vi "_LC Get Status.vi"(8 "Stream#":u8) -> (0 "error out":errorcluster, 1 "Error":bool, 2 "Ready":bool, 3 "LC Status":string, 4 "StatusIndicator":u16(ring)=1 caption="Status Indicator")   [LabVIEW 2015]
uses:
  Type/_LC Command.ctl
  _Global LC Driver.vi
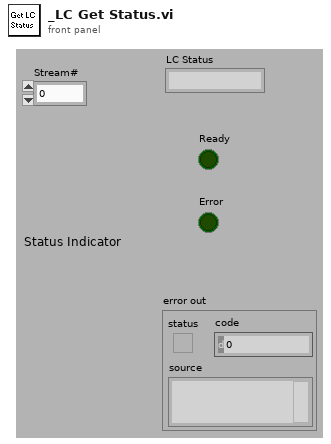
[diagram p1: front panel]
types:
  T1 = typedef "_LC Command.ctl" = enum16{"No Command", "Initialize", "Get Configuration", "Get Status", "Get LC Method Contents", "Oven OnOff", "Pump OnOFF", "Rinse Autosampler", "Run Sample", "Set EnvParameters", "Set Method", "Start Equilibration", "Stop Run", "Get LastError", "Clear Error", "Close"}
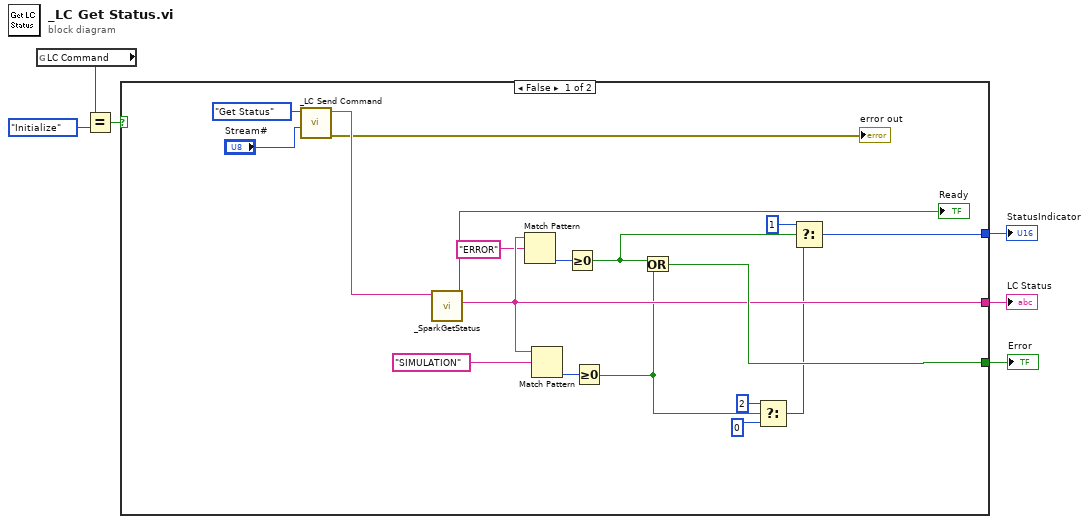
[diagram p0: block diagram]
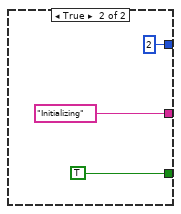
[diagram p2: hidden frame]
diagram:
  n1 = global read "_Global LC Driver.vi" "LC Command"() -> (w3:T1)
  n2 = Equal?(x=w3, y=_LC_Command."Initialize") -> (x = y?=w2:bool)
  n3 = case shown="False" w2 {
    tunnel: [w23 TRUE] -> w6
    tunnel: [w22 "Initializing" ("LCStatus")] -> w5
    tunnel: [w17 u16 2 ("LC Connection")] -> w1
    frame False {
      n4 = call "_LC Send Command.vi"("Stream#"="Stream#", "Command"=_LC_Command."Get Status") -> ("error out"=→"error out":errorcluster, "Reply"=w20:string)  [unwired: 8 in]
      n5 = call "_SparkGetStatus.vi"("SparkStatus"=w20) -> ("LCStatus"=w22:string, "Ready"=→"Ready":bool)  [unwired: 3 in, 6 out]
      n6 = Match Pattern(string=w22, regular expression="ERROR" ("format string")) -> (offset past match=w14:i32)  [unwired: 4 out]
      n7 = Match Pattern(string=w22, regular expression="SIMULATION" ("format string")) -> (offset past match=w16:i32)  [unwired: 4 out]
      n8 = Greater Or Equal To 0?(x=w14) -> (x >= 0?=w12:bool)
      n9 = Greater Or Equal To 0?(x=w16) -> (x >= 0?=w10:bool)
      n10 = Or(x=w12, y=w10) -> (x .or. y?=w23:bool)
      n11 = Select(t=u16 2 ("LC Connection"), s=w10, f=u16 0 ("LC Connection")) -> (s? t:f=w7:u16)
      n12 = Select(t=u16 1 ("LC Connection"), s=w12, f=w7) -> (s? t:f=w17:u16)
    }
    frame True {
    }
  }
  "LC Status" <- w5
  "Error" <- w6
  "StatusIndicator" <- w1
